vi "Process.vi"(8 "error in (no error)":errorcluster, 11 "RemoteControl":refnum<class "RemoteControl.lvclass">) -> (0 "error out":errorcluster, 3 "RemoteControl out":refnum<class "RemoteControl.lvclass">)   [LabVIEW 2019, in "RemoteControl.lvclass"]
doc: "---------------------------------------------------------------\nJKI State Machine Objects™\nhttp://jki.net/state-machine-objects/\nCopyright (C) 2005-2015, JKI <info@jki.net>\nALL RIGHTS RESERVED"
uses:
  RemoteControl.lvclass
  <vilib>/JKI/JKI SMO/SMO/SMO.lvclass
  Typedefs/Message--Cluster.ctl
  Typedefs/RC Process Type--Enum.ctl
  <vilib>/JKI/JKI SMO/SMO/Typedefs/SMOState --Enum.ctl
  <vilib>/JKI/JKI SMO/SMO/Typedefs/Reserve State--Enum.ctl
  <vilib>/JKI/JKI SMO/SMO/Typedefs/Public Events.ctl
  <vilib>/ErrorRing/Error Ring.xnode
  <userlib>/LevyLab/Configuration/Debug.lvlib
  C:/Program Files (x86)/National Instruments/LabVIEW 2019/vi.lib/JKI/JKI SMO/SMO/SMO.lvclass
panel:
  out "Process Type":string
  out "Message Out":string
  out "Message In":string
  in  "delay response":bool
  in  "create server error":bool
  in  "create listener error":bool
  out "State History":string
  out "Connections":i32
  in  "Message Timing?":bool
  in  "timeout (ms) [500]":i32=500
  in  "stop":bool
  # "Remote Control"
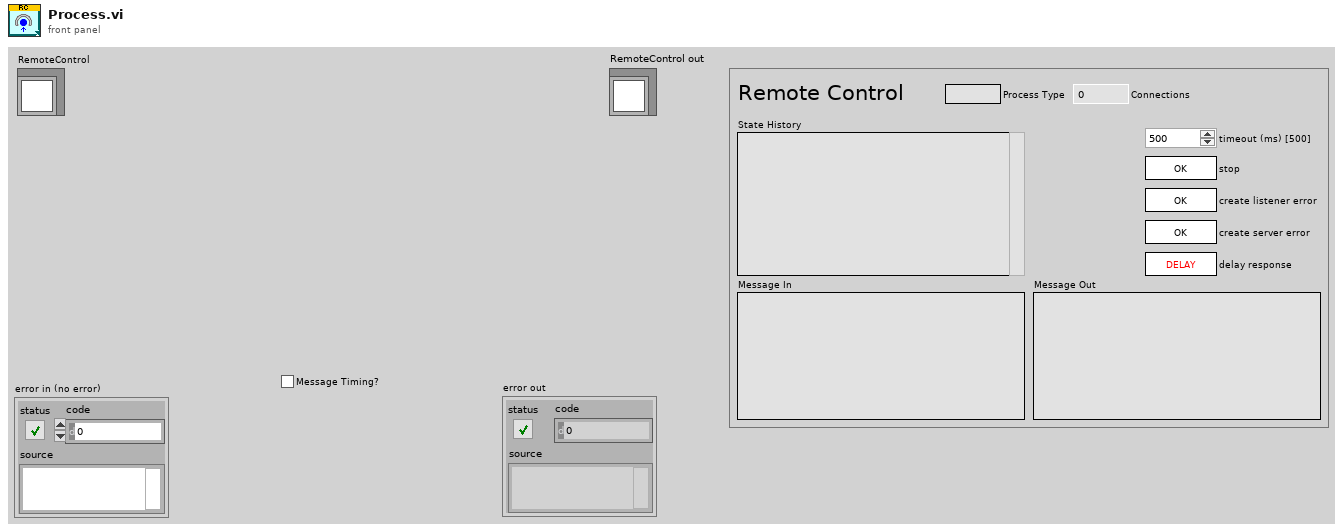
[diagram p1: front panel]
types:
  T1 = enum32{"invalid app kind", "Development System", "Run Time System", "Student Edition", "Embedded LabVIEW", "Evaluation", "Custom"}
  T2 = enum32{"Invalid", "Standard", "Closed", "Hidden", "Minimized", "Maximized"}
  T3 = typedef "RemoteControl.lvclass/Message--Cluster.ctl" = cluster{"Command":string, "Data":variant, "ID":string}
  T4 = typedef "RemoteControl.lvclass/RC Process Type--Enum.ctl" = enum16{"Listener", "Server", "Client"}
  T5 = cluster{"Current VI Reference":refnum<vi>, "Close Panel on Exit?":bool, "Last Error":cluster{"error":errorcluster, "previous state":string, "remaining states":string}, "Shutdown?":bool}
  T6 = typedef "RemoteControl.lvclass/PrivateEvents--RemoteControl.Configure.ctl" = cluster{"address":string, "Port":u16, "AllowedRemote":string, "Commands":string[], "timeout":i32}
  T7 = cluster{"Core":cluster{"Current VI Reference":refnum<vi>, "Close Panel on Exit?":bool, "Last Error":cluster{"error":errorcluster, "previous state":string, "remaining states":string}, "Shutdown?":bool}, "SelfRef":refnum<class "RemoteControl.lvclass">, "Listener":refnum<class "RemoteControl.lvclass">, "RC Process Type":T4, "Configure":T6, "Messages (in)":T3[], "Messages (out)":T3[], "state":enum16{"waiting", "processing"}, "to":i32, "UI Behavior":string, "wait":i32}
  T8 = typedef "Debug.lvlib/Attribute.Debug.lvclass/DebugBehavior.ctl" = enum16{"Normal", "Debug"}
  T9 = typedef "smo.lvlib/SMO.lvclass/Public Events.ctl" = cluster{"Error":refnum<user-event>, "State":refnum<user-event>, "Reserve State":refnum<user-event>}
  T10 = typedef "smo.lvlib/SMO.lvclass/Protected Events.ctl" = cluster{"StopProcesses":refnum<user-event>, "AbortProcesses":refnum<user-event>, "Config Changed":refnum<user-event>, "Dependency":refnum<user-event>}
  T11 = typedef "RemoteControl.lvclass/PrivateEvents--Cluster.ctl" = cluster{"Configure":refnum<user-event>, "SendMessageToProcess":refnum<user-event>}
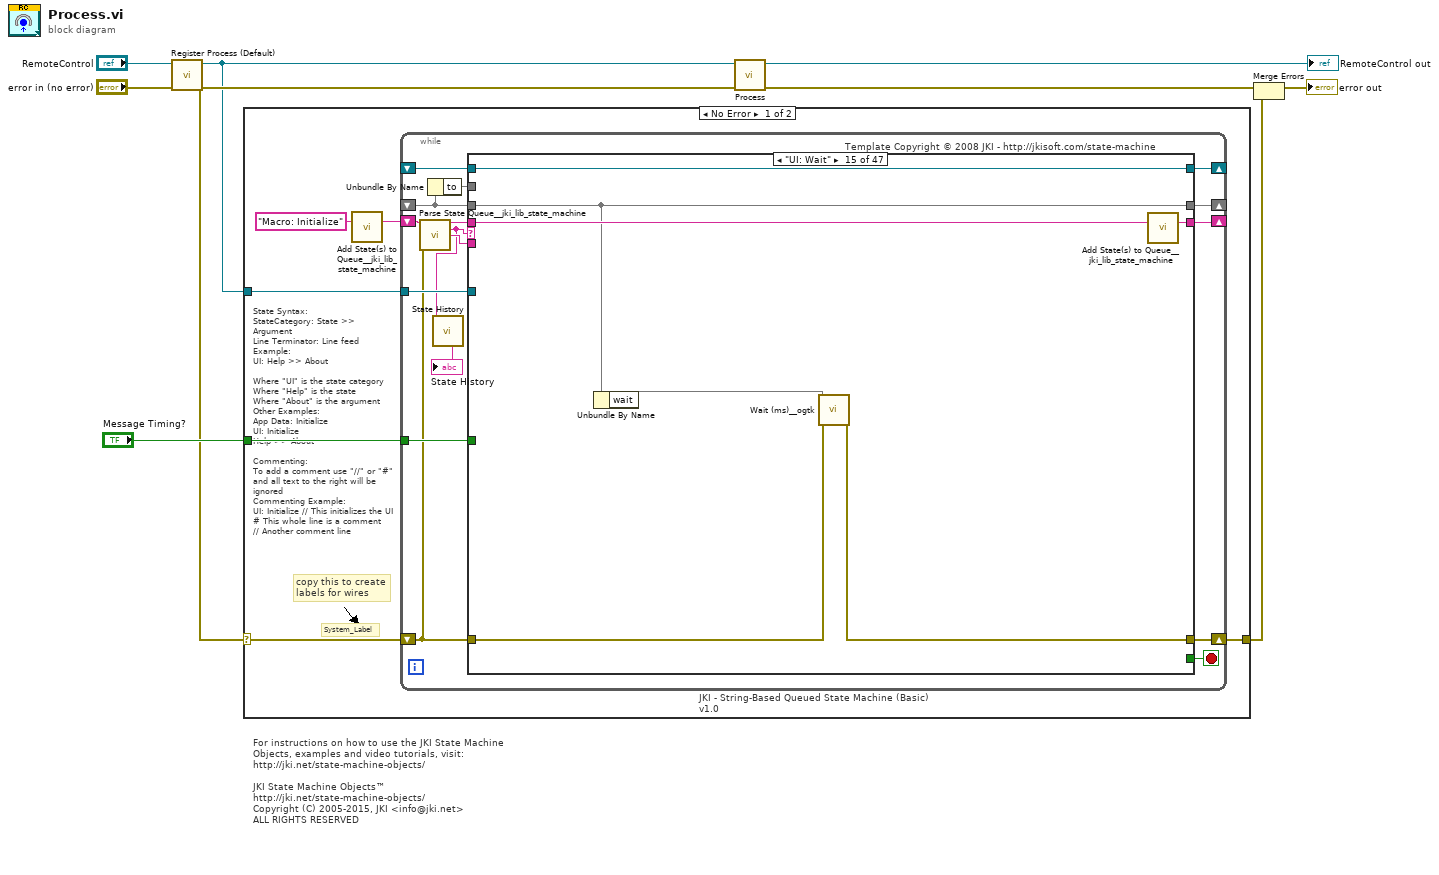
[diagram p0: block diagram]
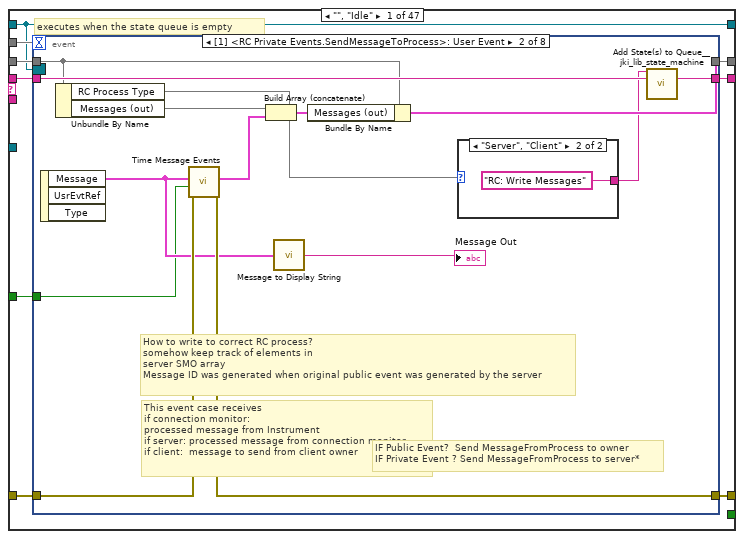
[diagram p2: hidden frame]
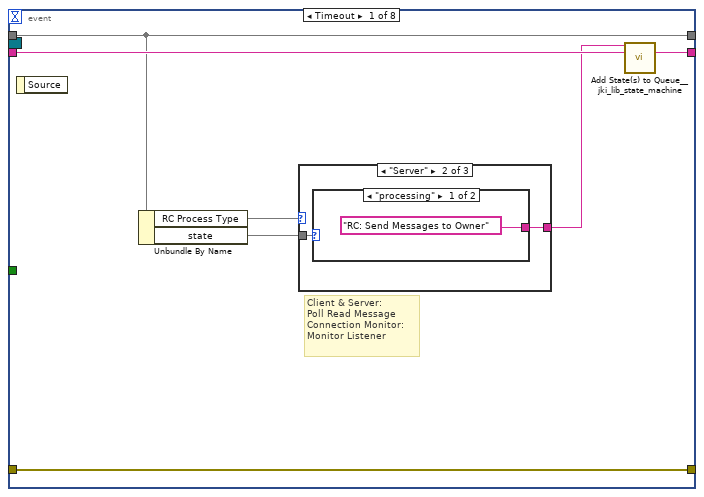
[diagram p3: hidden frame]
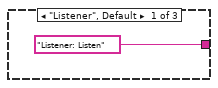
[diagram p4: hidden frame]
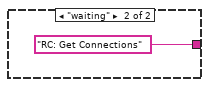
[diagram p5: hidden frame]
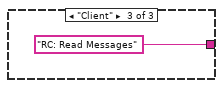
[diagram p6: hidden frame]
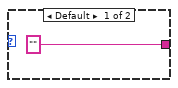
[diagram p7: hidden frame]
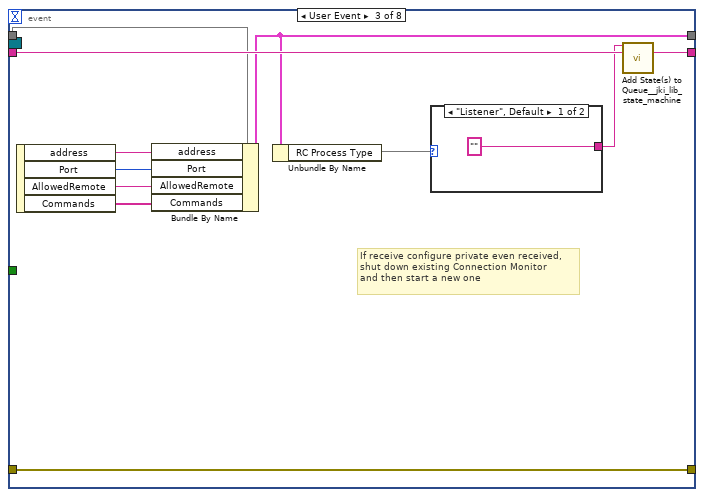
[diagram p8: hidden frame]
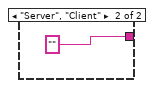
[diagram p9: hidden frame]
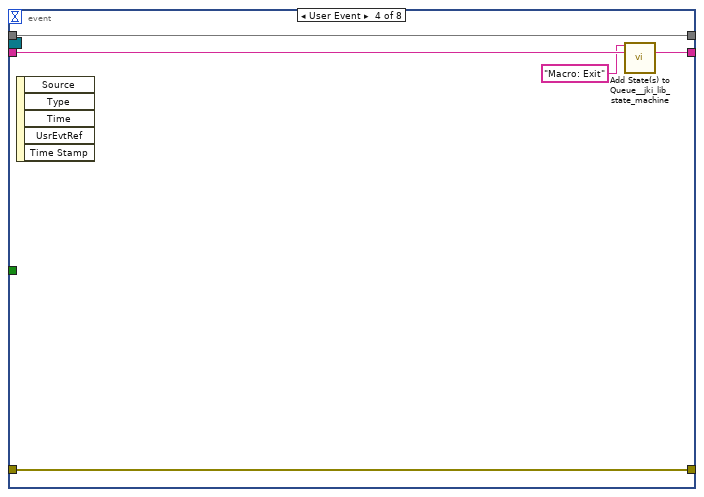
[diagram p10: hidden frame]
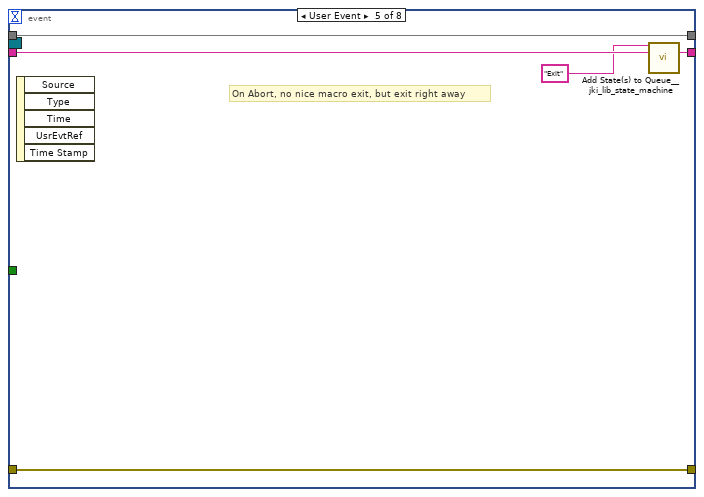
[diagram p11: hidden frame]
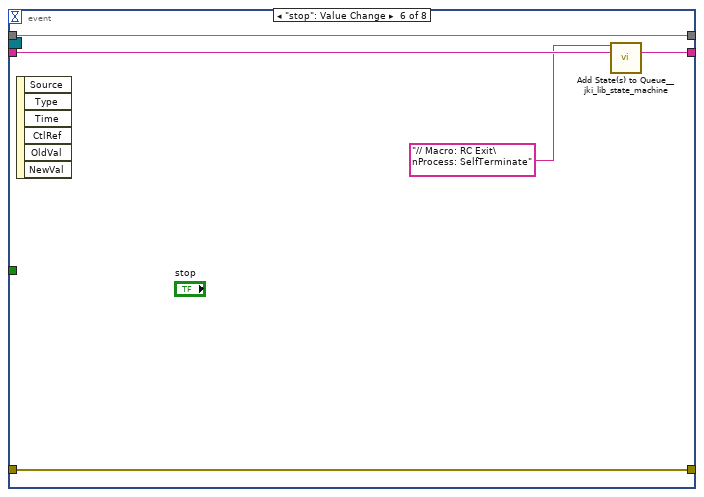
[diagram p12: hidden frame]
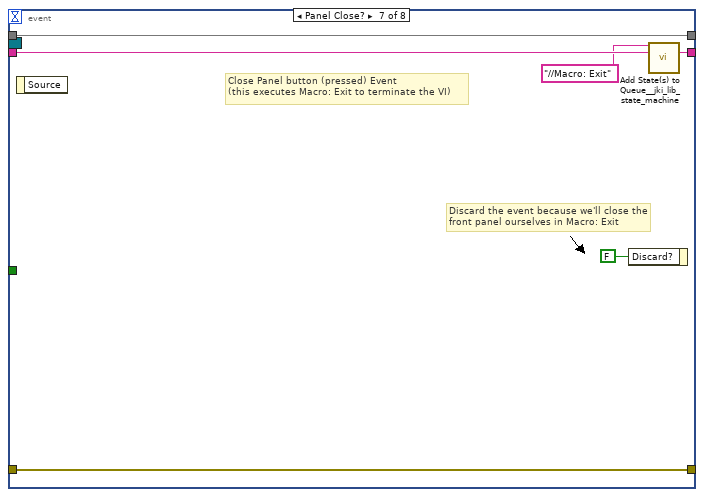
[diagram p13: hidden frame]
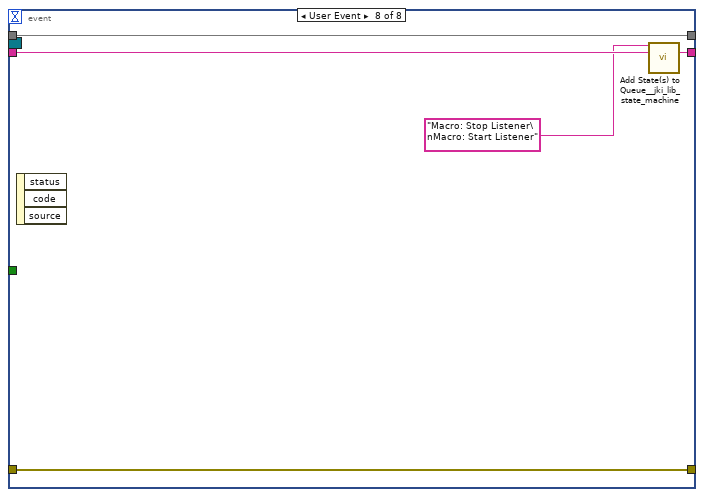
[diagram p14: hidden frame]
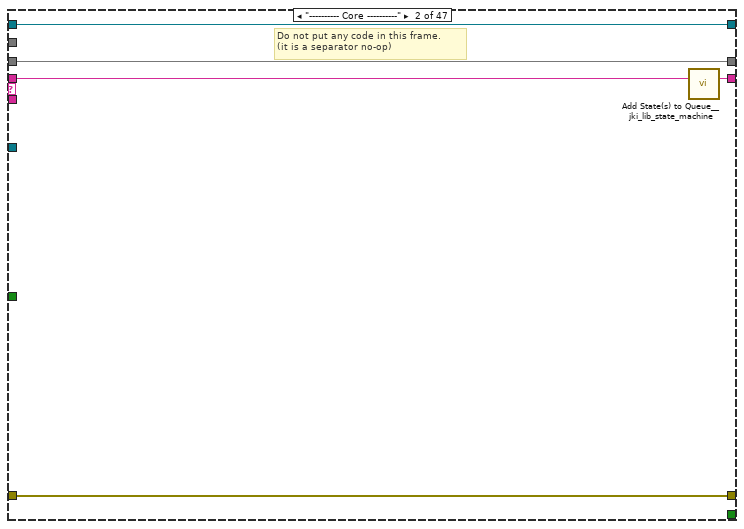
[diagram p15: hidden frame]
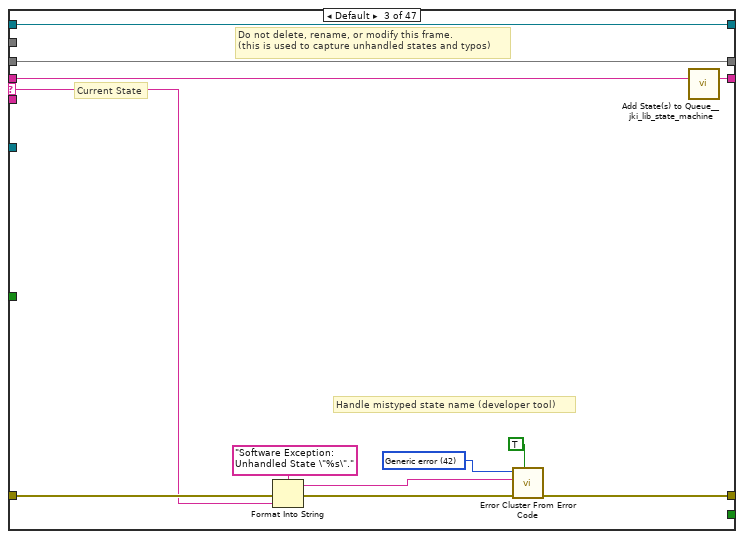
[diagram p16: hidden frame]
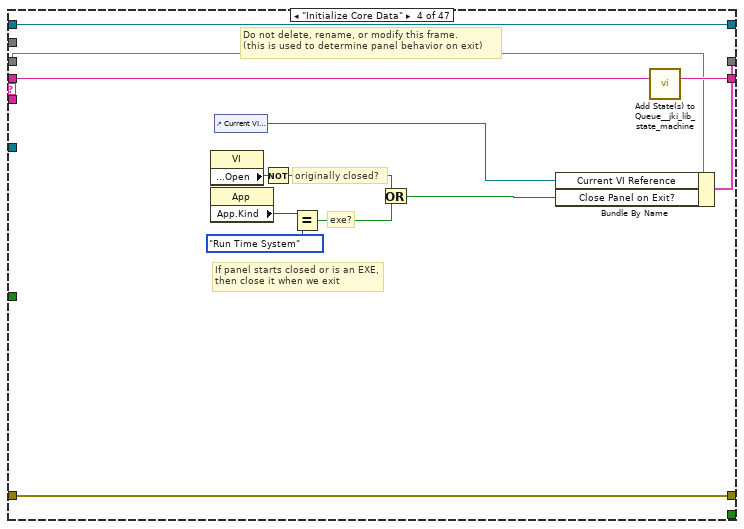
[diagram p17: hidden frame]
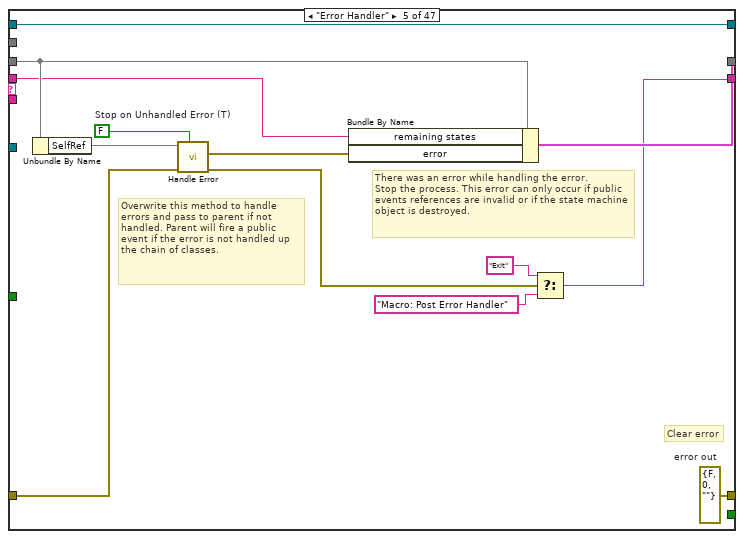
[diagram p18: hidden frame]
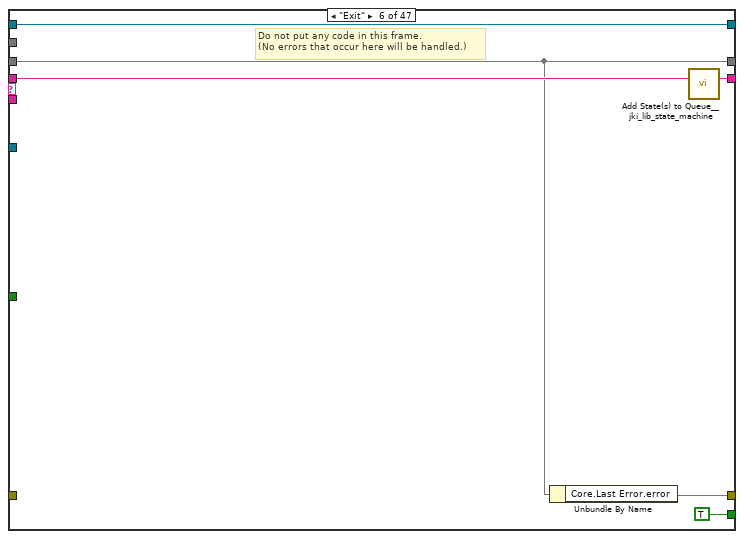
[diagram p19: hidden frame]
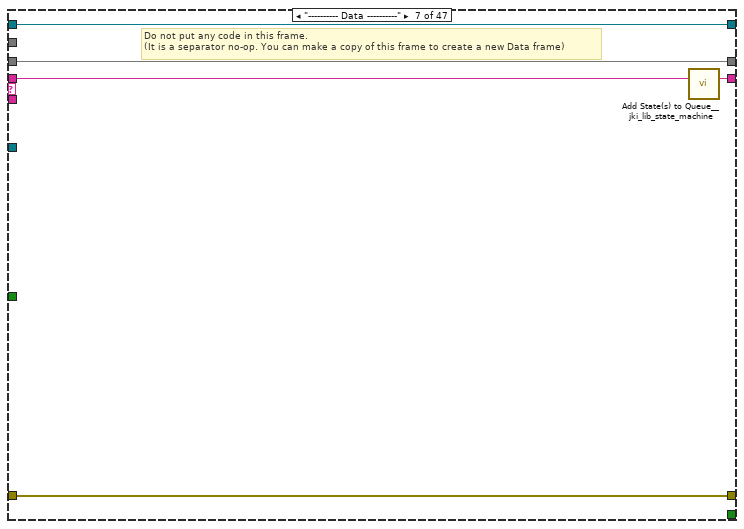
[diagram p20: hidden frame]
diagram:
  # "For instructions on how to use the JKI State Machine Objects, examples and video tutorials, visit:\nhttp://jki.net/state-machine-objects/\n\nJKI State Machine Objects™\nhttp://jki.net/state-machine-objects/\nCopyright (C) 2005-2015, JKI <info@jki.net>\nALL RIGHTS RESERVED"
  n1 = call <vilib>:"Register Process (Default).vi"("error in (no error)"="error in (no error)", "SMO"="RemoteControl") -> ("error out"=w3:errorcluster, "SelfRef"=w2:refnum<class "RemoteControl.lvclass">)  [unwired: 8 in]
  n2 = case shown="No Error" w3 {
    selector: w3 -> [w12 w673]
    tunnel: w2 -> [w13 _]
    tunnel: [w11 w673] -> w5
    tunnel: "Message Timing?" -> [w10 _]
    frame No Error {
      # "State Syntax:\nStateCategory: State >> Argument\nLine Terminator: Line feed\nExample:\nUI: Help >> About\n\nWhere \"UI\" is the state category\nWhere \"Help\" is the state\nWhere \"About\" is the argument\nOther Examples:\nApp Data: Initialize\nUI: Initialize\nHelp >> About\n\nCommenting:\nTo add a comment use \"//\" or \"#\" and all text to the right will be ignored\nCommenting Example:\nUI: Initialize // This initializes the UI\n# This whole line is a comment\n// Another comment line"
      # "copy this to create labels for wires"
      # "System_Label"
      n3 = call <vilib>:"Add State(s) to Queue__jki_lib_state_machine.vi"("State(s) in (\"\")"="Macro: Initialize") -> ("States Out"=w15:string)  [unwired: 14 in]
      n4 = while "JKI - String-Based Queued State Machine (Basic) v1.0" {
        shift-right: [w26] -> _
        shift-left: _ -> [w18]
        shift-right: [w28] -> w11
        shift-left: w12 -> [w21]
        shift-right: [w19] -> _
        shift-left: w15 -> [w29]
        tunnel: w13 -> [w25]
        shift-right: [w24] -> _
        shift-left: _ -> [w23]
        tunnel: w10 -> [w22]
        stop <- w27 stop-if-true
        # "Template Copyright © 2008 JKI - http://jkisoft.com/state-machine"
        n5 = call <vilib>:"Parse State Queue__jki_lib_state_machine.vi"("State Queue"=w29, "Error In (no error)"=w21) -> ("Remaining States"=w31:string, "Current State"=w20:string, "Arguments"=w30:string)  [unwired: 11 in]
        n6 = Unbundle By Name(w18) -> ("to"=w17)
        n7 = call "State History.vi"("Current State"=w20) -> ("History"=→"State History":string)  [unwired: 10 in]
        n8 = case shown="\"UI: Wait\"" w20 {
          selector: w20 -> [_ _ w115 _ _ _ _ _ _ _ _ _ _ _ _ _ _ _ _ _ _ _ _ _ _ _ _ _ _ _ _ _ _ _ _ _ _ _ _ _ _ _ _ _ _ _ _]
          tunnel: w31 -> [w40 w113 w119 w138 w141 w157 w162 w179 w195 w210 w215 w225 w236 w252 w284 w289 w301 w309 w316 w328 w339 w348 w365 w387 w392 w403 w412 w417 w431 w445 w451 w456 w465 w486 w519 w553 w576 w589 w598 w607 w614 w625 w636 w641 w650 w662 w672]
          tunnel: w30 -> [_ _ _ _ _ _ _ _ _ _ _ _ w230 w247 _ _ _ _ _ _ _ _ _ _ _ _ _ _ _ _ _ _ _ _ _ _ _ _ _ _ _ _ _ _ _ _ _]
          tunnel: [w37 w111 w121 w135 w150 w152 w160 w171 w181 w207 w213 w217 w231 w245 w278 w287 w299 w307 w312 w320 w331 w346 w363 w385 w390 w395 w405 w415 w425 w440 w447 w452 w462 w474 w511 w546 w568 w584 w590 w599 w610 w620 w631 w637 w645 w651 w667] -> w28
          tunnel: [w39 w112 w118 w137 w144 w156 w161 w178 w194 w209 w214 w224 w235 w251 w283 w288 w300 w308 w315 w327 w338 w347 w364 w386 w391 w402 w411 w416 w430 w444 w450 w455 w464 w485 w518 w552 w575 w588 w597 w606 w613 w624 w635 w640 w649 w661 w671] -> w19
          tunnel: [_ _ _ _ _ TRUE _ _ _ _ _ _ _ _ _ _ _ _ _ _ _ _ _ _ _ _ _ _ _ _ _ _ _ _ _ _ _ _ _ _ _ _ _ _ _ _ _] -> w27
          tunnel: [w35 w110 w117 w136 w148 w153 w159 w175 w183 w206 w212 w222 w234 w249 w281 w286 w291 w303 w310 w324 w335 w343 w361 w376 w389 w400 w409 w414 w429 w443 w449 w454 w457 w483 w515 w544 w571 w585 w594 w601 w608 w617 w628 w639 w643 w658 w666] -> w26
          tunnel: w17 -> [w34 _ _ _ _ _ _ _ _ _ _ _ _ _ _ _ _ _ _ _ _ _ _ _ _ _ _ _ _ _ _ _ _ _ _ _ _ _ _ _ _ _ _ _ _ _ _]
          tunnel: w25 -> [_ _ _ _ _ _ _ w167 _ _ _ _ _ _ _ _ _ _ _ _ _ _ _ _ _ _ _ _ _ _ _ _ _ _ _ _ _ _ _ _ _ _ _ _ _ _ _]
          tunnel: [w33 w109 w114 w126 w151 w154 w158 w177 w193 w205 w211 w223 w233 w246 w282 w285 w298 w306 w314 w326 w337 w345 w362 w381 w388 w401 w410 w413 w428 w442 w448 w453 w463 w484 w517 w551 w574 w587 w596 w605 w612 w623 w634 w638 w648 w660 w670] -> w24
          tunnel: w23 -> [w33 w109 w114 w126 w151 w154 w158 w177 w193 w205 w211 w223 w233 w246 w282 w285 w298 w306 w314 w326 w337 w345 w362 w381 w388 w401 w410 w413 _ w438 w448 w453 w463 w484 w517 w551 w574 w587 w596 w605 w612 w623 w634 w638 w648 w660 w670]
          tunnel: w22 -> [w32 _ _ _ _ _ _ _ _ _ _ _ _ _ _ _ _ _ _ _ _ _ _ _ _ _ _ _ _ _ _ _ w460 _ w516 w549 _ _ _ _ _ _ _ _ _ _ _]
          tunnel: w21 -> [w36 w111 w120 w135 w146 _ w160 w171 w180 w208 w213 w216 w232 w250 w279 w287 w299 w307 w312 w321 w332 w346 w363 w385 w390 w396 w406 w415 w426 w441 w447 w452 w459 w480 w501 w547 w569 w577 w591 w600 w611 w621 w632 w637 w646 w655 w668]
          tunnel: w18 -> [w38 w110 w117 w129 w149 w153 w159 _ w182 w206 w212 w222 w234 w249 w281 w286 w291 w303 w310 w324 w335 w343 w358 w375 w389 w400 w404 w414 w429 w443 w449 w454 w457 w482 w503 w545 w572 w586 w595 w602 w608 w618 w629 w639 w642 w659 w666]
          frame "", "Idle" {
            # "executes when the state queue is empty"
            n9 = event shown="[1] <RC Private Events.SendMessageToProcess>: User Event" {
              selector: w33 -> [_ _ _ _ _ _ _ _]
              dyn-events: _ -> [_ _ _ _ _ _ _ _]
              timeout: w34 -> [_ _ _ _ _ _ _ _]
              tunnel: w40 -> [w47 w67 w79 w87 w92 w96 w103 w108]
              tunnel: [w46 w66 w78 w86 w91 w97 w102 w107] -> w39
              tunnel: w38 -> [w42 w63 w77 w84 w89 w95 w100 w105]
              tunnel: [w45 w60 w80 w85 w90 w93 w101 w106] -> w37
              tunnel: w36 -> [w45 w59 w80 w85 w90 w93 w101 w106]
              tunnel: [w42 w65 w75 w84 w89 w95 w100 w105] -> w35
              tunnel: w32 -> [_ w54 _ _ _ _ _ _]
              event Timeout {
                # "Client & Server:\nPoll Read Message\nConnection Monitor:\nMonitor Listener"
                n10 = event-data() -> ()  [unwired: 1 in, 1 out]
                n11 = Unbundle By Name(w42) -> ("RC Process Type"=w43, "state"=w41)
                n12 = case shown="\"Server\"" w43 {
                  tunnel: ["Listener: Listen" ("State(s) in Front (\"\")") w50 "RC: Read Messages" ("State(s) in Front (\"\")")] -> w44
                  tunnel: w41 -> [_ w49 _]
                  frame "Listener", Default {
                  }
                  frame "Server" {
                    n13 = case shown="\"processing\"" w49 {
                      tunnel: ["RC: Send Messages to Owner" ("State(s) in Front (\"\")") "RC: Get Connections" ("State(s) in Front (\"\")")] -> w50
                      frame "processing" {
                      }
                      frame "waiting" {
                      }
                    }
                  }
                  frame "Client" {
                  }
                }
                n14 = call <vilib>:"Add State(s) to Queue__jki_lib_state_machine.vi"("State(s) in Front (\"\")"=w44, "State(s) in (\"\")"=w47) -> ("States Out"=w46:string)  [unwired: 13 in]
              }
              event User Event {
                # "IF Public Event?  Send MessageFromProcess to owner\nIF Private Event ? Send MessageFromProcess to server*"
                # "How to write to correct RC process?\nsomehow keep track of elements in\nserver SMO array\nMessage ID was generated when original public event was generated by the server"
                # "This event case receives\nif connection monitor:\nprocessed message from Instrument\nif server: processed message from connection monitor\nif client:  message to send from client owner"
                n15 = event-data() -> ("Message"=w56:T3)  [unwired: 1 in, 2 out]
                n16 = Unbundle By Name(w63) -> ("RC Process Type"=w58, "Messages (out)"=w62)
                n17 = call "Time Message Events.vi"("error in (no error)"=w59, "Debug Mode"=w54, "Message in"=w56) -> ("error out"=w60:errorcluster, "Message out"=w57:T3)  [unwired: 5 in, 2 out]
                n18 = Build Array (concatenate)(w62, w57) -> (w61:T3[])
                n19 = call "Message to Display String.vi"("Message"=w56) -> ("message string"=→"Message Out":string)
                n20 = Bundle By Name(cluster=w63, "Messages (out)"=w61) -> (w65:cluster{})
                n21 = case shown="\"Server\", \"Client\"" w58 {
                  tunnel: ["" ("State(s) in Front (\"\")") "RC: Write Messages" ("State(s) in Front (\"\")")] -> w64
                  frame Default {
                  }
                  frame "Server", "Client" {
                  }
                }
                n22 = call <vilib>:"Add State(s) to Queue__jki_lib_state_machine.vi"("State(s) in Front (\"\")"=w64, "State(s) in (\"\")"=w67) -> ("States Out"=w66:string)  [unwired: 13 in]
              }
              event User Event {
                # "If receive configure private even received,\nshut down existing Connection Monitor \nand then start a new one"
                n23 = event-data() -> ("address"=w70:string, "Port"=w71:u16, "AllowedRemote"=w72:string, "Commands"=w73:string[])  [unwired: 1 in]
                n24 = Bundle By Name(cluster=w77, "address"=w70, "Port"=w71, "AllowedRemote"=w72, "Commands"=w73) -> (w75:cluster{})
                n25 = Unbundle By Name(w75) -> ("RC Process Type"=w76)
                n26 = case shown="\"Listener\", Default" w76 {
                  tunnel: ["" ("State(s) in Front (\"\")") "" ("State(s) in Front (\"\")")] -> w74
                  frame "Listener", Default {
                  }
                  frame "Server", "Client" {
                  }
                }
                n27 = call <vilib>:"Add State(s) to Queue__jki_lib_state_machine.vi"("State(s) in Front (\"\")"=w74, "State(s) in (\"\")"=w79) -> ("States Out"=w78:string)  [unwired: 13 in]
              }
              event User Event {
                n28 = event-data() -> ()  [unwired: 1 in, 5 out]
                n29 = call <vilib>:"Add State(s) to Queue__jki_lib_state_machine.vi"("State(s) in Front (\"\")"="Macro: Exit", "State(s) in (\"\")"=w87) -> ("States Out"=w86:string)  [unwired: 13 in]
              }
              event User Event {
                # "On Abort, no nice macro exit, but exit right away"
                n30 = event-data() -> ()  [unwired: 1 in, 5 out]
                n31 = call <vilib>:"Add State(s) to Queue__jki_lib_state_machine.vi"("State(s) in Front (\"\")"="Exit", "State(s) in (\"\")"=w92) -> ("States Out"=w91:string)  [unwired: 13 in]
              }
              event "stop": Value Change {
                n32 = event-data() -> ()  [unwired: 1 in, 6 out]
                n33 = call <vilib>:"Add State(s) to Queue__jki_lib_state_machine.vi"("State(s) in Front (\"\")"="// Macro: RC Exit\nProcess: SelfTerminate" ("State(s) in Front (\"\")"), "State(s) in (\"\")"=w96) -> ("States Out"=w97:string)  [unwired: 13 in]
              }
              event Panel Close? {
                # "Discard the event because we'll close the front panel ourselves in Macro: Exit"
                # "Close Panel button (pressed) Event\n(this executes Macro: Exit to terminate the VI)"
                n34 = event-data() -> ()  [unwired: 1 in, 1 out]
                n35 = event-data("Discard?"=FALSE) -> ()  [unwired: 1 in, 1 out]
                n36 = call <vilib>:"Add State(s) to Queue__jki_lib_state_machine.vi"("State(s) in Front (\"\")"="//Macro: Exit", "State(s) in (\"\")"=w103) -> ("States Out"=w102:string)  [unwired: 13 in]
              }
              event User Event {
                n37 = event-data() -> ()  [unwired: 1 in, 3 out]
                n38 = call <vilib>:"Add State(s) to Queue__jki_lib_state_machine.vi"("State(s) in Front (\"\")"="Macro: Stop Listener\nMacro: Start Listener", "State(s) in (\"\")"=w108) -> ("States Out"=w107:string)  [unwired: 13 in]
              }
            }
          }
          frame "---------- Core ----------" {
            # "Do not put any code in this frame.\n(it is a separator no-op)"
            n39 = call <vilib>:"Add State(s) to Queue__jki_lib_state_machine.vi"("State(s) in (\"\")"=w113) -> ("States Out"=w112:string)  [unwired: 14 in]
          }
          frame Default {
            w124 = 42 items=["No error", "Argument error", "Memory is full", "Out of zone", "End of file", "File already open", "Generic file I/O error", "File not found", "File permission error", "Disk is full", "Duplicate path", "Too many files open", "System feature not enabled", "Resource file not found", "Cannot add resource", "Resource not found", "Image not found", "Image memory error", "Pen does not exist", "Config type invalid", "Config token not found", "Config parse error", "Config memory error", "Bad external code format", "Bad external code offset", "External code not present", "Null window", "Destroy window error", "Null menu", "Print aborted", "Bad print record", "Print driver error", "Windows error during printing", "Memory error during printing", "Print dialog error", "Generic print error", "Invalid device refnum", "Device not found", "Device parameter error", "Device unit error", "Cannot open device", "Device call aborted", "Generic error", "Cancelled by user", "Object ID too low", "Object ID too high", "Object not in heap", "Unknown heap", "Unknown object (invalid DefProc)", "Unknown object (DefProc not in table)", "Message out of range", "Invalid (null) method", "Unknown message", "Manager call not supported", "Bad address", "Network operation in progress", "Network operation timed out", "Connection is busy", "Network attribute not supported", "Network error", "Address in use", "System out of memory", "Connection aborted", "Connection refused", "Not connected", "Already connected", "Connection closed", "Initialization error (interapplication manager)", "Bad occurrence", "Wait on unbound occurrence handler", "Occurrence queue overflow", "Datalog type conflict", "Unused", "Unrecognized type (interapplication manager)", "Memory corrupt", "Failed to make temporary DLL", "Old CIN version", "Drag socket not found", "Failed to load drop-object", "Failed to register OLE object", "Failed to release OLE object", "Format specifier type mismatch", "Unknown format specifier", "Too few format specifiers", "Too many format specifiers", "Scan failed", "Newer CIN version", "Error converting to variant", "Runtime menu error", "Password tampered", "Variant attribute not found", "Incompatible variant data type", "Event data is not available", "Event Store is not present", "Occurrence is not found", "Event Queue is not created", "Event info is not available", "Refnum passed is NULL", "Error retrieving Class GUID", "Error retrieving CoClass GUID", "Error retrieving TypeLib GUID.", "Bad built application magic bytes.", "Specific driver is different from the specific driver associated with the Logical Name.", "There is no session opened to the class driver.", "Max Error", "MAX - Error with config objects", "MAX - Error loading configuration", "MAX - Group not supported"]
            # "Current State"
            # "Do not delete, rename, or modify this frame.\n(this is used to capture unhandled states and typos)"
            # "Handle mistyped state name (developer tool)"
            n40 = Format Into String(format string="Software Exception: Unhandled State \"%s\"." ("message"), error in=w120, w115) -> (resulting string=w123:string, error out=w122:errorcluster)  [unwired: 1 in]
            n41 = call <vilib>:"Error Cluster From Error Code.vi"("show call chain? (False)"=TRUE, "error in (no error)"=w122, "error message (\"\")"=w123, "error code (0)"=w124) -> ("error out"=w121:errorcluster)  [unwired: 5 in]
            n42 = call <vilib>:"Add State(s) to Queue__jki_lib_state_machine.vi"("State(s) in (\"\")"=w119) -> ("States Out"=w118:string)  [unwired: 14 in]
          }
          frame "Initialize Core Data" {
            # "Do not delete, rename, or modify this frame.\n(this is used to determine panel behavior on exit)"
            # "originally closed?"
            # "exe?"
            # "If panel starts closed or is an EXE, then close it when we exit"
            n43 = property class="VI"() -> ("Front Panel.Open"=w134:bool)  [unwired: 2 in, 2 out]
            n44 = property class="App"() -> ("App.Kind"=w133:T1)  [unwired: 2 in, 2 out]
            n45 = control-ref of="Current VI Reference"() -> (w127:refnum<vi>)
            n46 = Not(x=w134) -> (.not. x?=w131:bool)
            n47 = Equal?(x=w133, y=T1."Run Time System" ("Application:Kind")) -> (x = y?=w130:bool)
            n48 = Or(x=w131, y=w130) -> (x .or. y?=w128:bool)
            n49 = Bundle By Name(cluster=w129, "Current VI Reference"=w127, "Close Panel on Exit?"=w128) -> (w136:cluster{})
            n50 = call <vilib>:"Add State(s) to Queue__jki_lib_state_machine.vi"("State(s) in (\"\")"=w138) -> ("States Out"=w137:string)  [unwired: 14 in]
          }
          frame "Error Handler" {
            w147 = FALSE  # Stop on Unhandled Error (T)
            w150 = errorcluster {"status"=FALSE, "code"=0, "source"=""}  # error out
            # "There was an error while handling the error.\nStop the process. This error can only occur if public events references are invalid or if the state machine object is destroyed."
            # "Clear error"
            # "Overwrite this method to handle errors and pass to parent if not handled. Parent will fire a public event if the error is not handled up the chain of classes."
            n51 = Unbundle By Name(w149) -> ("SelfRef"=w145)
            n52 = call-dynamic "Handle Error.vi"("Stop on Unhandled Error (T)"=w147, "error in"=w146, "SMO"=w145) -> ("handling error"=w142:errorcluster, "Unhandled error"=w143:errorcluster)  [unwired: 6 in, 1 out]
            n53 = Bundle By Name(cluster=w149, "remaining states"=w141, "error"=w143) -> (w148:cluster{})
            n54 = Select(t="Exit", s=w142, f="Macro: Post Error Handler") -> (s? t:f=w144:string)
          }
          frame "Exit" {
            # "Do not put any code in this frame.\n(No errors that occur here will be handled.)"
            n55 = Unbundle By Name(w153) -> ("Core.Last Error.error"=w152)
            n56 = call <vilib>:"Add State(s) to Queue__jki_lib_state_machine.vi"("State(s) in (\"\")"=w157) -> ("States Out"=w156:string)  [unwired: 14 in]
          }
          frame "---------- Data ----------" {
            # "Do not put any code in this frame.\n(It is a separator no-op. You can make a copy of this frame to create a new Data frame)"
            n57 = call <vilib>:"Add State(s) to Queue__jki_lib_state_machine.vi"("State(s) in (\"\")"=w162) -> ("States Out"=w161:string)  [unwired: 14 in]
          }
          frame "Data: Initialize" {
            w164 = ""  # UI Behavior
            w163 = 0  # wait
            w168 = 10  # to
            w169 = enum16{"waiting", "processing"}."waiting"  # state
            w170 = refnum<class "RemoteControl.lvclass"> refnum  # Listener
            w172 = T3[] []  # Messages (out)
            w173 = T3[] []  # Messages (in)
            w176 = T5 {"Current VI Reference"=refnum, "Close Panel on Exit?"=FALSE, "Last Error"={"error"={"status"=FALSE, "code"=0, "source"=""}, "previous state"="", "remaining states"=""}, "Shutdown?"=FALSE}  # Core
            # "do not delete - used by framework"
            # "Initialize the shift-register data, here.\n(data names are defined by what you wire into the bundle function)"
            n58 = Unbundle By Name(w167) -> ("RC Process Type"=w165:T4, "Configure"=w174:T6)
            n59 = Format Into String(w165) -> (resulting string=→"Process Type":string)  [unwired: 3 in, 1 out]
            n60 = Bundle("Core"=w176, "SelfRef"=w167, "Listener"=w170, "RC Process Type"=w165, "Configure"=w174, "Messages (in)"=w173, "Messages (out)"=w172, "state"=w169, "to"=w168, "UI Behavior"=w164, "wait"=w163) -> (w175:T7)  [unwired: 1 in]
            n61 = call <vilib>:"Add State(s) to Queue__jki_lib_state_machine.vi"("State(s) in (\"\")"=w179) -> ("States Out"=w178:string)  [unwired: 14 in]
          }
          frame "Data: Debug" {
            # "exe?"
            # "If pane is an EXE, then close it when we exit"
            # "Data: Debug\n(get debug behavior, determine UI and determine shutdown behavior)"
            n62 = Unbundle By Name(w182) -> ("Core.Close Panel on Exit?"=w185, "SelfRef"=w192)
            n63 = property class="App"() -> ("App.Kind"=w188:T1)  [unwired: 2 in, 2 out]
            n64 = Equal?(x=w188, y=T1."Run Time System" ("Application:Kind")) -> (x = y?=w184:bool)
            n65 = call <userlib>:"Get Debug Mode.vi"("error in (no error)"=w180, "SMO"=w192) -> ("error out"=w181:errorcluster, "Behavior"=w191:T8)  [unwired: 7 in, 1 out]
            n66 = case shown="\"Debug\"" w191 {
              tunnel: ["Close" "Open"] -> w190
              tunnel: [u32 0 ("wait") u32 1000 ("wait")] -> w189
              tunnel: [w196 w199] -> w186
              tunnel: w185 -> [w196 _]
              tunnel: w184 -> [_ w201]
              frame "Normal", Default {
                # "respect core.close"
              }
              frame "Debug" {
                # "keep panel open\nunless exe"
                n67 = Or(x=w201, y=FALSE) -> (x .or. y?=w199:bool)
              }
            }
            n68 = Bundle By Name(cluster=w182, "Close Panel on Exit?"=w186, "UI Behavior"=w190, "wait"=w189) -> (w183:cluster{})
            n69 = call <vilib>:"Add State(s) to Queue__jki_lib_state_machine.vi"("State(s) in (\"\")"=w195) -> ("States Out"=w194:string)  [unwired: 14 in]
          }
          frame "Data: Cleanup" {
            # "Cleanup any data and references, here.\n(this is called automatically, by the Macro: Exit)"
            n70 = Unbundle By Name(w206) -> ("Core.Current VI Reference"=w204)
            n71 = Close Reference(reference=w204, error in (no error)=w208) -> (error out=w207:errorcluster)
            n72 = call <vilib>:"Add State(s) to Queue__jki_lib_state_machine.vi"("State(s) in (\"\")"=w210) -> ("States Out"=w209:string)  [unwired: 14 in]
          }
          frame "---------- UI ----------" {
            # "Do not put any code in this frame.\n(It is a separator no-op. You can make a copy of this frame to create a new UI frame)"
            n73 = call <vilib>:"Add State(s) to Queue__jki_lib_state_machine.vi"("State(s) in (\"\")"=w215) -> ("States Out"=w214:string)  [unwired: 14 in]
          }
          frame "UI: Initialize" {
            # "Initialize the User Interface, here.\n(this is called automatically, by the Macro: Init)"
            n74 = Unbundle By Name(w222) -> ("RC Process Type"=w221)
            n75 = case shown="\"Server\", Default" w221 {
              tunnel: [FALSE TRUE] -> w220
              tunnel: [TRUE FALSE] -> w219
              frame "Listener" {
              }
              frame "Server", Default {
              }
            }
            n76 = call <userlib>:"Fit VI window to Largest Dec__ogtk.vi"("error in (no error)"=w216, "border spacing (2 px)"=0) -> ("error out"=w217:errorcluster)  [unwired: 4 in, 1 out]
            n77 = property on="create server error" class="Bool (strict)"("Visible"=w220) -> ()  [unwired: 2 in, 2 out]
            n78 = property on="create listener error" class="Bool (strict)"("Visible"=w219) -> ()  [unwired: 2 in, 2 out]
            n79 = call <vilib>:"Add State(s) to Queue__jki_lib_state_machine.vi"("State(s) in (\"\")"=w225) -> ("States Out"=w224:string)  [unwired: 14 in]
          }
          frame "UI: Cursor Set" {
            # "Argument"
            # "Initialize the User Interface, here.\n(this is called automatically, by the Macro: Init)"
            n80 = disable-structure shown="Default" {
              disable-tunnel: w232 -> [w237 w240]
              disable-tunnel: [w237 w239] -> w231
              disable-tunnel: w230 -> [_ w238]
              frame condition #0 {
              }
              frame condition #1 (active) {
                n81 = case shown="\"Idle\", Default" w238 {
                  tunnel: w240 -> [w242 w244]
                  tunnel: [w241 w243] -> w239
                  frame "Idle", Default {
                    n82 = call <vilib>:"Unset Busy.vi"("error in (no error)"=w242) -> ("error out"=w241:errorcluster)  [unwired: 10 in]
                  }
                  frame "Busy" {
                    n83 = call <vilib>:"Set Busy.vi"("error in (no error)"=w244) -> ("error out"=w243:errorcluster)  [unwired: 9 in, 1 out]
                  }
                }
              }
            }
            n84 = call <vilib>:"Add State(s) to Queue__jki_lib_state_machine.vi"("State(s) in (\"\")"=w236) -> ("States Out"=w235:string)  [unwired: 14 in]
          }
          frame "UI: Front Panel State" {
            # "Argument"
            # "Set Front Panel Open or Closed\n(Usage: \"UI: Front Panel State >> Open|Close\")"
            n85 = Unbundle By Name(w249) -> ("Core.Current VI Reference"=w248)
            n86 = disable-structure shown="Default" {
              disable-tunnel: w250 -> [w256 w277]
              disable-tunnel: [w255 w277] -> w245
              disable-tunnel: w248 -> [w254 _]
              disable-tunnel: w247 -> [w253 _]
              frame condition #0 (active) {
                n87 = case shown="\"Close\"" w253 {
                  tunnel: w256 -> [w260 w271]
                  tunnel: [w261 w272] -> w255
                  tunnel: w254 -> [_ _]
                  frame "Open", Default {
                    n88 = property class="VI"(error in=w260) -> (reference out=w258:refnum<vi>, error out=w259:errorcluster, "FP.State"=w257:T2)  [unwired: 1 in]
                    n89 = case shown="\"Closed\"" w257 {
                      tunnel: [w264 w267] -> w261
                      tunnel: w259 -> [w263 w267]
                      tunnel: w258 -> [w262 _]
                      frame "Closed" {
                        n90 = invoke class="VI" method="FP.Open"(reference=w262, error in=w263, "Activate"=TRUE, "State"=T2."Standard") -> (error out=w264:errorcluster)  [unwired: 1 in, 4 out]
                      }
                      frame Default {
                      }
                    }
                  }
                  frame "Close" {
                    n91 = property class="VI"(error in=w271) -> (reference out=w269:refnum<vi>, error out=w270:errorcluster, "FP.State"=w268:T2)  [unwired: 1 in]
                    n92 = case shown="Default" w268 {
                      tunnel: [w273 w276] -> w272
                      tunnel: w270 -> [w273 w275]
                      tunnel: w269 -> [_ w274]
                      frame "Invalid", "Closed" {
                      }
                      frame Default {
                        n93 = invoke class="VI" method="FP.Close"(reference=w274, error in=w275) -> (error out=w276:errorcluster)  [unwired: 1 in, 2 out]
                      }
                    }
                  }
                }
              }
              frame condition #1 {
              }
            }
            n94 = call <vilib>:"Add State(s) to Queue__jki_lib_state_machine.vi"("State(s) in (\"\")"=w252) -> ("States Out"=w251:string)  [unwired: 14 in]
          }
          frame "UI: Wait" {
            n95 = Unbundle By Name(w281) -> ("wait"=w280)
            n96 = call <userlib>:"Wait (ms)__ogtk.vi"("error in (no error)"=w279, "milliseconds to wait"=w280) -> ("error out"=w278:errorcluster)  [unwired: 8 in, 1 out]
            n97 = call <vilib>:"Add State(s) to Queue__jki_lib_state_machine.vi"("State(s) in (\"\")"=w284) -> ("States Out"=w283:string)  [unwired: 14 in]
          }
          frame "---------- Macro ----------" {
            # "Do not put any code in this frame.\n(It is a separator no-op. You can make a copy of this frame to create a new Macro frame)"
            n98 = call <vilib>:"Add State(s) to Queue__jki_lib_state_machine.vi"("State(s) in (\"\")"=w289) -> ("States Out"=w288:string)  [unwired: 14 in]
          }
          frame "Macro: Initialize" {
            # "Initialization Macro\n(This is called once, when the VI starts)"
            n99 = call <vilib>:"Add State(s) to Queue__jki_lib_state_machine.vi"("State(s) in Front (\"\")"="UI: Initialize", "State(s) in (\"\")"="UI: Front Panel State >> Close", "State(s) at Back (\"\")"="Macro: Debug\nMacro: RC Initialize") -> ("States Out"=w292:string)  [unwired: 12 in]
            n100 = call <vilib>:"Add State(s) to Queue__jki_lib_state_machine.vi"("State(s) in Front (\"\")"="Data: Initialize\nInitialize Core Data\nEvents: Register", "State(s) in (\"\")"="Process: Sync", "State(s) at Back (\"\")"=w292) -> ("States Out"=w296:string)  [unwired: 12 in]
            n101 = call <vilib>:"Add State(s) to Queue__jki_lib_state_machine.vi"("State(s) in Front (\"\")"=w296, "State(s) in (\"\")"=w301) -> ("States Out"=w300:string)  [unwired: 13 in]
          }
          frame "Macro: Debug" {
            n102 = Unbundle By Name(w303) -> ("UI Behavior"=w305)
            n103 = Format Into String(format string="Data: Debug\nUI: Front Panel State >> %s\nUI: Wait" ("State(s) in Front (\"\")"), w305) -> (resulting string=w302:string)  [unwired: 2 in, 1 out]
            n104 = call <vilib>:"Add State(s) to Queue__jki_lib_state_machine.vi"("State(s) in Front (\"\")"=w302, "State(s) in (\"\")"=w309) -> ("States Out"=w308:string)  [unwired: 13 in]
          }
          frame "Macro: RC Initialize" {
            n105 = Unbundle By Name(w310) -> ("RC Process Type"=w313)
            n106 = case shown="\"Server\"" w313 {
              tunnel: ["Listener: Start Listener" ("State(s) in Front (\"\")") "Macro: Start Listener\nRC: Open Server Connection" ("State(s) in Front (\"\")") "RC: Open Client Connection" ("State(s) in Front (\"\")")] -> w311
              frame "Listener", Default {
              }
              frame "Server" {
              }
              frame "Client" {
              }
            }
            n107 = call <vilib>:"Add State(s) to Queue__jki_lib_state_machine.vi"("State(s) in Front (\"\")"=w311, "State(s) in (\"\")"=w316) -> ("States Out"=w315:string)  [unwired: 13 in]
          }
          frame "Macro: Start Listener" {
            n108 = Unbundle By Name(w324) -> ("SelfRef"=w323)
            n109 = call <vilib>:"Get LV Class Name.vi"("error in (no error)"=w321, "object"=w323) -> ("error out"=w320:errorcluster, "class name"=w322:string)  [unwired: 8 in]
            n110 = case shown="\"RemoteControl.STM.lvclass\"" w322 {
              tunnel: ["" ("State(s) in Front (\"\")") "RC: Create Listener SMO\nEvents: Register Listener SMO\nRC: Start Listener SMO" ("State(s) in Front (\"\")")] -> w325
              frame Default {
              }
              frame "RemoteControl.STM.lvclass" {
              }
            }
            n111 = call <vilib>:"Add State(s) to Queue__jki_lib_state_machine.vi"("State(s) in Front (\"\")"=w325, "State(s) in (\"\")"=w328) -> ("States Out"=w327:string)  [unwired: 13 in]
          }
          frame "Macro: Stop Listener" {
            n112 = Unbundle By Name(w335) -> ("SelfRef"=w334)
            n113 = call <vilib>:"Get LV Class Name.vi"("error in (no error)"=w332, "object"=w334) -> ("error out"=w331:errorcluster, "class name"=w333:string)  [unwired: 8 in]
            n114 = case shown="\"RemoteControl.STM.lvclass\"" w333 {
              tunnel: ["" ("State(s) in Front (\"\")") "RC: Stop Listener SMO\nRC: Destroy Listener SMO" ("State(s) in Front (\"\")")] -> w336
              frame Default {
              }
              frame "RemoteControl.STM.lvclass" {
              }
            }
            n115 = call <vilib>:"Add State(s) to Queue__jki_lib_state_machine.vi"("State(s) in Front (\"\")"=w336, "State(s) in (\"\")"=w339) -> ("States Out"=w338:string)  [unwired: 13 in]
          }
          frame "Macro: RC Exit" {
            n116 = Unbundle By Name(w343) -> ("RC Process Type"=w342)
            n117 = case shown="\"Server\"" w342 {
              tunnel: ["Listener: Stop Listener" ("State(s) in Front (\"\")") "Macro: Stop Listener\nRC: Close Connection" ("State(s) in Front (\"\")")] -> w344
              frame "Listener", Default {
              }
              frame "Server" {
              }
            }
            n118 = call <vilib>:"Add State(s) to Queue__jki_lib_state_machine.vi"("State(s) in Front (\"\")"=w344, "State(s) in (\"\")"=w348) -> ("States Out"=w347:string)  [unwired: 13 in]
          }
          frame "Macro: Post Error Handler" {
            # "Clear Last Error?"
            n119 = Unbundle By Name(w358) -> ("Core.Last Error.error"=w353)
            n120 = Unbundle By Name(w358) -> ("RC Process Type"=w354, "Core.Last Error.remaining states"=w357, "Core.Shutdown?"=w356)
            n121 = case shown="False" FALSE {
              tunnel: w353 -> [w366 _]
              tunnel: [w366 _] -> w351
              frame False {
              }
              frame True {
              }
            }
            n122 = case shown="False" w356 {
              tunnel: w357 -> [_ w372]
              tunnel: [w367 w371] -> w355
              tunnel: w354 -> [w368 _]
              frame False {
                # "These are the remaining states (at the moment the error occured). States can be altered according to business logic."
                # "NOT SHUTTING DOWN"
                n123 = case shown="\"Server\"" w368 {
                  tunnel: ["" ("State(s) in Front (\"\")") "Macro: RC Exit\nMacro: RC Initialize" ("State(s) in Front (\"\")")] -> w367
                  frame Default {
                    # "If Listener, owner will restart\nListener process"
                  }
                  frame "Server" {
                  }
                }
              }
              frame True {
                # "Developer can decide to alter the states but should be aware that during the shutdown process, there are certain states that must be run for the SMO to properly shut itself (and this process) down. As such, one can add states to perform additional clean-ups, but should append the remaining state to be executed."
                # "SHUTTING DOWN"
                n124 = call <vilib>:"Add State(s) to Queue__jki_lib_state_machine.vi"("State(s) in (\"\")"=w372) -> ("States Out"=w371:string)  [unwired: 14 in]
              }
            }
            n125 = Bundle By Name(cluster=w358, "error"=w351, "Messages (out)"=T3[] [], "state"=enum16{"waiting", "processing"}."waiting") -> (w361:cluster{})
            n126 = call <vilib>:"Add State(s) to Queue__jki_lib_state_machine.vi"("State(s) in Front (\"\")"=w355, "State(s) in (\"\")"=w365) -> ("States Out"=w364:string)  [unwired: 13 in]
          }
          frame "Macro: Exit" {
            # "Exit Macro\n(This is called once, when the VI exits)"
            n127 = Unbundle By Name(w375) -> ("Core.Close Panel on Exit?"=w377)
            n128 = Bundle By Name(cluster=w375, "Shutdown?"=TRUE ("Core.Shutdown?")) -> (w376:cluster{})
            n129 = Select(t="UI: Front Panel State >> Close", s=w377, f="") -> (s? t:f=w383:string)
            n130 = call <vilib>:"Add State(s) to Queue__jki_lib_state_machine.vi"("State(s) in Front (\"\")"="Macro: RC Exit", "State(s) at Back (\"\")"="Data: Cleanup\nEvents: Unregister\nProcess: Sync\nExit") -> ("States Out"=w378:string)  [unwired: 13 in]
            n131 = call <vilib>:"Add State(s) to Queue__jki_lib_state_machine.vi"("State(s) in (\"\")"=w383, "State(s) at Back (\"\")"=w378) -> ("States Out"=w382:string)  [unwired: 13 in]
            n132 = call <vilib>:"Add State(s) to Queue__jki_lib_state_machine.vi"("State(s) in Front (\"\")"=w382, "State(s) in (\"\")"=w387) -> ("States Out"=w386:string)  [unwired: 13 in]
          }
          frame "---------- Process ----------" {
            # "Template Separator\n(You can make a copy of, or modify, this frame)"
            n133 = call <vilib>:"Add State(s) to Queue__jki_lib_state_machine.vi"("State(s) in (\"\")"=w392) -> ("States Out"=w391:string)  [unwired: 14 in]
          }
          frame "Process: Sync" {
            n134 = Unbundle By Name(w400) -> ("SelfRef"=w393)
            n135 = call <vilib>:"WaitOnProcessSync.vi"("error in (no error)"=w396, "SMO"=w393) -> ("error out"=w395:errorcluster, "Don't run?"=w399:bool)  [unwired: 7 in, 1 out]
            n136 = Select(t="Data: Cleanup\nEvents: Unregister\nExit", s=w399, f="") -> (s? t:f=w394:string)
            n137 = call <vilib>:"Add State(s) to Queue__jki_lib_state_machine.vi"("State(s) in Front (\"\")"=w394, "State(s) in (\"\")"=w403) -> ("States Out"=w402:string)  [unwired: 13 in]
          }
          frame "Process: SelfTerminate" {
            n138 = Unbundle By Name(w404) -> ("SelfRef"=w408)
            n139 = call <vilib>:"SelfTerminate.vi"("error in (no error)"=w406, "SMO in"=w408) -> ("error out"=w405:errorcluster, "SMO out"=w407:refnum<class "SMO.lvclass">)  [unwired: 8 in]
            n140 = Bundle By Name(cluster=w404, "SelfRef"=w407) -> (w409:cluster{})
            n141 = call <vilib>:"Add State(s) to Queue__jki_lib_state_machine.vi"("State(s) in (\"\")"=w412) -> ("States Out"=w411:string)  [unwired: 14 in]
          }
          frame "---------- Events ----------" {
            # "Template Separator\n(You can make a copy of, or modify, this frame)"
            n142 = call <vilib>:"Add State(s) to Queue__jki_lib_state_machine.vi"("State(s) in (\"\")"=w417) -> ("States Out"=w416:string)  [unwired: 14 in]
          }
          frame "Events: Register" {
            w419 = T9 {"Error"=refnum, "State"=refnum, "Reserve State"=refnum}  # Listener Public Events
            # "Expand to add\nmore events"
            n143 = Unbundle By Name(w429) -> ("SelfRef"=w418)
            n144 = call <vilib>:"GetProtectedEvents.vi"("SMO"=w418) -> ("error out"=w423:errorcluster, "SMO Protected Events"=w427:T10, "SMO out"=w421:refnum<class "SMO.lvclass">)  [unwired: 8 in]
            n145 = call "RemoteControl.GetPrivateEvents.vi"("RemoteControl"=w421) -> ("error out"=w422:errorcluster, "RC Private Events"=w420:T11)  [unwired: 8 in, 1 out]
            n146 = register-events(w427, w420, w419) -> (reference out=w428:refnum<event-registration>, error out=w424:errorcluster)  [unwired: 2 in]
            n147 = Merge Errors(w422, w426, w424, w423) -> (w425:errorcluster)
            n148 = call <vilib>:"Add State(s) to Queue__jki_lib_state_machine.vi"("State(s) in (\"\")"=w431) -> ("States Out"=w430:string)  [unwired: 14 in]
          }
          frame "Events: Register Listener SMO" {
            w436 = T9 {"Error"=refnum, "State"=refnum, "Reserve State"=refnum}  # Listener Public Events
            n149 = Unbundle By Name(w443) -> ("Listener"=w437)
            n150 = call <vilib>:"GetPublicEvents.vi"("SMO"=w437) -> ("error out"=w435:errorcluster, "Public Events"=w433:T9)  [unwired: 8 in, 1 out]
            n151 = Variant To Data(error in=w435, type=w436, Variant=w433) -> (data=w432:T9, error out=w434:errorcluster)
            n152 = register-events(reference=w438, w432) -> (reference out=w442:refnum<event-registration>, error out=w439:errorcluster)  [unwired: 3 in]
            n153 = Merge Errors(w441, w439, w434) -> (w440:errorcluster)
            n154 = call <vilib>:"Add State(s) to Queue__jki_lib_state_machine.vi"("State(s) in (\"\")"=w445) -> ("States Out"=w444:string)  [unwired: 14 in]
          }
          frame "Events: Unregister" {
            n155 = Unregister For Events(event registration refnum=w448, error in=w447) -> (error out=w446:errorcluster)
            n156 = call <vilib>:"Clear Errors.vi"("error in (no error)"=w446) -> ()  [unwired: 5 in, 2 out]
            n157 = call <vilib>:"Add State(s) to Queue__jki_lib_state_machine.vi"("State(s) in (\"\")"=w451) -> ("States Out"=w450:string)  [unwired: 14 in]
          }
          frame "---------- RC ----------" {
            # "Template Separator\n(You can make a copy of, or modify, this frame)"
            n158 = call <vilib>:"Add State(s) to Queue__jki_lib_state_machine.vi"("State(s) in (\"\")"=w456) -> ("States Out"=w455:string)  [unwired: 14 in]
          }
          frame "RC: Send Messages to Owner" {
            # "This loop will run # times equal to messages in the queue"
            # "Send Message to Owner to be processed\n(Send a message to the instrument to be processed)"
            n159 = Unbundle By Name(w457) -> ("SelfRef"=w461, "Messages (in)"=w458)
            n160 = for {
              tunnel: w461 -> [w467]
              tunnel: w460 -> [w471]
              tunnel: w458 -> [w466]
              tunnel: w459 -> [w470]
              tunnel: [w473] -> w462
              n161 = call "Time Message Events.vi"("error in (no error)"=w470, "Debug Mode"=w471, "Message in"=w466, "RemoteControl"=w467) -> ("error out"=w472:errorcluster, "Message out"=w469:T3, "RemoteControl out"=w468:refnum<class "RemoteControl.lvclass">)  [unwired: 4 in, 1 out]
              n162 = call "RemoteControl.SendMessageFromProcess.vi"("error in (no error)"=w472, "Message"=w469, "RemoteControl"=w468) -> ("error out"=w473:errorcluster)  [unwired: 7 in, 1 out]
            }
            n163 = call <vilib>:"Add State(s) to Queue__jki_lib_state_machine.vi"("State(s) in (\"\")"=w465) -> ("States Out"=w464:string)  [unwired: 14 in]
          }
          frame "RC: Get Connections" {
            # "Here listen for new connections and then stop after timeout or if there's a new connection"
            n164 = Unbundle By Name(w482) -> ("SelfRef"=w481)
            n165 = call-dynamic "Get Connections.vi"("error in (no error)"=w480, "RemoteControl in"=w481) -> ("error out"=w475:errorcluster, "Number"=w478:i32, "RemoteControl out"=w479:refnum<class "RemoteControl.lvclass">)  [unwired: 7 in]
            "Connections" <- w478
            n166 = case shown="Default" w478 {
              selector: w478 -> [_ w493 _]
              tunnel: ["" ("State(s) in Front (\"\")") w492 "RC: Close Connection" ("State(s) in Front (\"\")")] -> w477
              frame 0 {
              }
              frame Default {
                # "read %d messages"
                n167 = Format Into String(format string="RC: Read Messages >> %d" ("State(s) in Front (\"\")"), w493) -> (resulting string=w492:string)  [unwired: 2 in, 1 out]
              }
              frame 100 {
              }
            }
            n168 = Bundle By Name(cluster=w482, "SelfRef"=w479) -> (w483:cluster{})
            n169 = xnode "Error Ring"() -> ()  [unwired: 1 out]
            n170 = case shown="True" "create server error" {
              tunnel: w475 -> [w488 _]
              tunnel: [w488 errorcluster {"status"=TRUE, "code"=-1001, "source"="Server error"} ("t")] -> w474
              frame False {
              }
              frame True {
                n171 = local write "create server error"(FALSE ("create listener error")) -> ()
              }
            }
            n172 = call <vilib>:"Add State(s) to Queue__jki_lib_state_machine.vi"("State(s) in Front (\"\")"=w477, "State(s) in (\"\")"=w486) -> ("States Out"=w485:string)  [unwired: 13 in]
          }
          frame "RC: Read Messages" {
            # "poll the number\nof open connections"
            # "Read Message over, eg TCP"
            # "If command is empty do not Send Message"
            n173 = Unbundle By Name(w503) -> ("SelfRef"=w502)
            n174 = Unbundle By Name(w503) -> ("to"=w509)
            n175 = call "Write Timeout.vi"("error in (no error)"=w501, "timeout (ms) [500]"="timeout (ms) [500]", "RemoteControl in"=w502) -> ("error out"=w500:errorcluster, "RemoteControl out"=w499:refnum<class "RemoteControl.lvclass">)  [unwired: 7 in]
            n176 = call-dynamic "Read Message.vi"("error in (no error)"=w500, "RemoteControl in"=w499) -> ("error out"=w507:errorcluster, "Data"=w504:string, "Command"=w505:string, "RemoteControl out"=w506:refnum<class "RemoteControl.lvclass">, "ID"=w508:string)  [unwired: 5 in]
            n177 = case shown="Default" w505 {
              selector: w505 -> [w523 _]
              tunnel: w508 -> [w526 _]
              tunnel: w507 -> [w528 w539]
              tunnel: [w528 w539] -> w511
              tunnel: w516 -> [_ _]
              tunnel: w506 -> [w524 w533]
              tunnel: w504 -> [w527 _]
              tunnel: [enum16{"waiting", "processing"}."processing" ("state") w538] -> w513
              tunnel: enum16{"waiting", "processing"}."waiting" ("state") -> [_ w538]
              tunnel: ["RC: Send Messages to Owner" ""] -> w512
              tunnel: [5000 w537] -> w510
              tunnel: w509 -> [_ w537]
              tunnel: [w525 w534] -> w497
              tunnel: [w524 w533] -> w496
              frame Default {
                n178 = To Variant(anything=w527) -> (Variant=w522:variant)
                n179 = Bundle By Name(cluster=T3 {"Command"="", "Data"=variant(string ""), "ID"=""} ("Message from Remote"), "Command"=w523, "Data"=w522, "ID"=w526) -> (w520:T3)
                n180 = call "Message to Display String.vi"("Message"=w520) -> ("message string"=→"Message In":string)
                n181 = Build Array(w520) -> (w525:T3[])
              }
              frame "" {
                # "Messages coming from TCP need to have command"
                n182 = Build Array(T3 {"Command"="", "Data"=variant(string ""), "ID"=""} ("Message out")) -> (w534:T3[])
              }
            }
            n183 = Bundle By Name(cluster=w503, "to"=w510, "state"=w513, "SelfRef"=w496, "Messages (in)"=w497) -> (w515:cluster{})
            n184 = call <vilib>:"Add State(s) to Queue__jki_lib_state_machine.vi"("State(s) in Front (\"\")"=w512, "State(s) in (\"\")"=w519) -> ("States Out"=w518:string)  [unwired: 13 in]
          }
          frame "RC: Write Messages" {
            # "After the loop completes\nempty the out queue"
            # "This loop will run # times equal to messages in the out queue"
            # "send Message over, eg. TCP"
            n185 = Unbundle By Name(w545) -> ("SelfRef"=w550, "Messages (out)"=w548)
            n186 = for {
              tunnel: w550 -> [w565]
              tunnel: w549 -> [w554]
              tunnel: w548 -> [w555]
              tunnel: [w557] -> w540
              tunnel: w547 -> [w563]
              tunnel: [w564] -> w546
              n187 = call "Time Message Events.vi"("error in (no error)"=w563, "Debug Mode"=w554, "Message in"=w555) -> ("error out"=w562:errorcluster, "Message out"=w556:T3)  [unwired: 5 in, 2 out]
              n188 = Unbundle By Name(w556) -> ("Command"=w558:string, "Data"=w559:variant, "ID"=w560:string)
              n189 = while {
                tunnel: w562 -> [w567]
                tunnel: [w567] -> w561
                stop <- "delay response" continue-if-true
              }
              n190 = call-dynamic "Send Message.vi"("ID"=w560, "error in (no error)"=w561, "Data"=w559, "Command"=w558, "RemoteControl in"=w565) -> ("error out"=w564:errorcluster, "RemoteControl out"=w557:refnum<class "RemoteControl.lvclass">)  [unwired: 5 in]
            }
            n191 = Bundle By Name(cluster=w545, "Messages (out)"=T3[] [], "state"=enum16{"waiting", "processing"}."waiting", "to"=5, "SelfRef"=w540) -> (w544:cluster{})
            n192 = call <vilib>:"Add State(s) to Queue__jki_lib_state_machine.vi"("State(s) in (\"\")"=w553) -> ("States Out"=w552:string)  [unwired: 14 in]
          }
          frame "RC: Close Connection" {
            # "Closes open server connections"
            # "call this on error 66, etc (when connection\ndrops). check these in error handler"
            n193 = Unbundle By Name(w572) -> ("SelfRef"=w573)
            n194 = call-dynamic "Close Connection.vi"("error in (no error)"=w569, "RemoteControl in"=w573) -> ("error out"=w568:errorcluster, "RemoteControl out"=w570:refnum<class "RemoteControl.lvclass">)  [unwired: 8 in]
            n195 = Bundle By Name(cluster=w572, "SelfRef"=w570) -> (w571:cluster{})
            n196 = call <vilib>:"Add State(s) to Queue__jki_lib_state_machine.vi"("State(s) in (\"\")"=w576) -> ("States Out"=w575:string)  [unwired: 14 in]
          }
          frame "RC: Create Listener SMO" {
            # "Create Listener SMO"
            n197 = Unbundle By Name(w586) -> ("SelfRef"=w579, "Configure"=w581)
            n198 = Bundle By Name(cluster=w579, "Configure"=w581, "RC Process Type"=RC_Process_Type--Enum."Listener") -> (w578:cluster{})
            n199 = call <vilib>:"Create.vi"("error in (no error)"=w577, "Subsystem Name (optional)"="Remote-Control-Listener" ("format string"), "SMO"=w578) -> ("error out"=w584:errorcluster, "SMO out"=w580:refnum<class "SMO.lvclass">)  [unwired: 6 in, 1 out]
            n200 = Bundle By Name(cluster=w586, "Listener"=w580) -> (w585:cluster{})
            n201 = call <vilib>:"Add State(s) to Queue__jki_lib_state_machine.vi"("State(s) in (\"\")"=w589) -> ("States Out"=w588:string)  [unwired: 14 in]
          }
          frame "RC: Start Listener SMO" {
            n202 = Unbundle By Name(w595) -> ("Listener"=w592)
            n203 = call <vilib>:"Start.vi"("error in (no error)"=w591, "SMO"=w592) -> ("error out"=w590:errorcluster, "SMO out"=w593:refnum<class "SMO.lvclass">)  [unwired: 8 in]
            n204 = Bundle By Name(cluster=w595, "Listener"=w593) -> (w594:cluster{})
            n205 = call <vilib>:"Add State(s) to Queue__jki_lib_state_machine.vi"("State(s) in (\"\")"=w598) -> ("States Out"=w597:string)  [unwired: 14 in]
          }
          frame "RC: Stop Listener SMO" {
            n206 = Unbundle By Name(w602) -> ("Listener"=w603)
            n207 = call <vilib>:"Stop.vi"("error in (no error)"=w600, "SMO"=w603) -> ("error out"=w599:errorcluster, "SMO out"=w604:refnum<class "SMO.lvclass">)  [unwired: 8 in]
            n208 = Bundle By Name(cluster=w602, "Listener"=w604) -> (w601:cluster{})
            n209 = call <vilib>:"Add State(s) to Queue__jki_lib_state_machine.vi"("State(s) in (\"\")"=w607) -> ("States Out"=w606:string)  [unwired: 14 in]
          }
          frame "RC: Destroy Listener SMO" {
            n210 = Unbundle By Name(w608) -> ("Listener"=w609)
            n211 = call <vilib>:"Destroy.vi"("error in (no error)"=w611, "SMO"=w609) -> ("error out"=w610:errorcluster)  [unwired: 9 in]
            n212 = call <vilib>:"Add State(s) to Queue__jki_lib_state_machine.vi"("State(s) in (\"\")"=w614) -> ("States Out"=w613:string)  [unwired: 14 in]
          }
          frame "RC: Open Client Connection" {
            n213 = Unbundle By Name(w618) -> ("SelfRef"=w622, "Configure.address"=w616, "Configure.Port"=w615)
            n214 = call-dynamic "Open Client Connection.vi"("error in (no error)"=w621, "Port"=w615, "address"=w616, "RemoteControl in"=w622) -> ("error out"=w620:errorcluster, "RemoteControl out"=w619:refnum<class "RemoteControl.lvclass">)  [unwired: 6 in]
            n215 = Bundle By Name(cluster=w618, "SelfRef"=w619) -> (w617:cluster{})
            n216 = call <vilib>:"Add State(s) to Queue__jki_lib_state_machine.vi"("State(s) in (\"\")"=w625) -> ("States Out"=w624:string)  [unwired: 14 in]
          }
          frame "RC: Open Server Connection" {
            n217 = Unbundle By Name(w629) -> ("SelfRef"=w633, "Configure.address"=w627, "Configure.Port"=w626)
            n218 = call-dynamic "Open Server Connection.vi"("error in (no error)"=w632, "Port"=w626, "address"=w627, "RemoteControl in"=w633) -> ("error out"=w631:errorcluster, "RemoteControl out"=w630:refnum<class "RemoteControl.lvclass">)  [unwired: 6 in]
            n219 = Bundle By Name(cluster=w629, "SelfRef"=w630) -> (w628:cluster{})
            n220 = call <vilib>:"Add State(s) to Queue__jki_lib_state_machine.vi"("State(s) in (\"\")"=w636) -> ("States Out"=w635:string)  [unwired: 14 in]
          }
          frame "---------- Listener ----------" {
            # "Template Separator\n(You can make a copy of, or modify, this frame)"
            n221 = call <vilib>:"Add State(s) to Queue__jki_lib_state_machine.vi"("State(s) in (\"\")"=w641) -> ("States Out"=w640:string)  [unwired: 14 in]
          }
          frame "Listener: Start Listener" {
            # "Start Asynchronous Listener"
            n222 = Unbundle By Name(w642) -> ("SelfRef"=w647)
            n223 = call-dynamic "Start Listener.vi"("error in (no error)"=w646, "RemoteControl in"=w647) -> ("error out"=w645:errorcluster, "RemoteControl out"=w644:refnum<class "RemoteControl.lvclass">)  [unwired: 8 in]
            n224 = Bundle By Name(cluster=w642, "SelfRef"=w644) -> (w643:cluster{})
            n225 = call <vilib>:"Add State(s) to Queue__jki_lib_state_machine.vi"("State(s) in (\"\")"=w650) -> ("States Out"=w649:string)  [unwired: 14 in]
          }
          frame "Listener: Listen" {
            n226 = Unbundle By Name(w659) -> ("SelfRef"=w656)
            n227 = call-dynamic "Listen.vi"("timeout ms (100) (wait forever: -1)"=1000, "error in (no error)"=w655, "RemoteControl"=w656) -> ("error out"=w652:errorcluster, "RemoteControl out"=w657:refnum<class "RemoteControl.lvclass">)  [unwired: 7 in]
            n228 = Bundle By Name(cluster=w659, "SelfRef"=w657) -> (w658:cluster{})
            n229 = case shown="True" "create listener error" {
              tunnel: w652 -> [w663 _]
              tunnel: [w663 errorcluster {"status"=TRUE, "code"=-1000, "source"="Listener error"} ("t")] -> w651
              frame False {
              }
              frame True {
                n230 = local write "create listener error"(FALSE ("create listener error")) -> ()
              }
            }
            n231 = call <vilib>:"Add State(s) to Queue__jki_lib_state_machine.vi"("State(s) in (\"\")"=w662) -> ("States Out"=w661:string)  [unwired: 14 in]
          }
          frame "Listener: Stop Listener" {
            # "Stop Asynchronous Listener \n(You can make a copy of, or modify, this frame)"
            n232 = Unbundle By Name(w666) -> ("SelfRef"=w669)
            n233 = call-dynamic "Stop Listener.vi"("error in (no error)"=w668, "RemoteControl in"=w669) -> ("error out"=w667:errorcluster)  [unwired: 8 in, 1 out]
            n234 = call <vilib>:"Add State(s) to Queue__jki_lib_state_machine.vi"("State(s) in (\"\")"=w672) -> ("States Out"=w671:string)  [unwired: 14 in]
          }
        }
      }
    }
    frame Error {
    }
  }
  n235 = call-parent "Process.vi"("error in"=w3, "SMO"=w2) -> ("error out"=w1:errorcluster, "SMO out"=→"RemoteControl out":refnum<class "RemoteControl.lvclass">)  [unwired: 8 in]
  n236 = Merge Errors(w1, w5) -> (→"error out":errorcluster)
